vi "Process.vi"(8 "error in":errorcluster, 11 "Inst UI.TSL210":refnum<class "Inst UI.TSL210.lvclass">) -> (0 "error out":errorcluster, 3 "Inst UI.TSL210 out":refnum<class "Inst UI.TSL210.lvclass">)   [LabVIEW 2019, in "Inst UI.TSL210.lvclass"]
doc: "---------------------------------------------------------------\nJKI State Machine Objects™\nhttp://jki.net/state-machine-objects/\nCopyright (C) 2005-2015, JKI <info@jki.net>\nALL RIGHTS RESERVEDJKI State Machine Objects (SMO) 1.0.0.5\nJKI - JKI\nCopyright (c) 2016, JKI"
uses:
  Inst UI.TSL210.lvclass
  C:/Program Files (x86)/National Instruments/LabVIEW 2019/vi.lib/JKI/JKI SMO/SMO/SMO.lvclass
  C:/Program Files (x86)/National Instruments/LabVIEW 2019/user.lib/LevyLab/Instrument Framework/SMOs/Instrument UI/Instrument UI.lvclass
  C:/Program Files (x86)/National Instruments/LabVIEW 2019/vi.lib/JKI/JKI SMO/SMO.UI/SMO.UI.lvclass
  Inst.TSL210/Typedefs/Inst.TSL210.getAll--Cluster.ctl
  Inst.TSL210/Inst.TSL210.lvclass
  C:/Program Files (x86)/National Instruments/LabVIEW 2019/user.lib/LevyLab/Instrument Framework/SMOs/Instrument/Instrument.lvclass
  Inst UI.TSL210.UI--Cluster.ctl
  Inst.TSL210/Typedefs/Inst.TSL210.Configuration--Cluster.ctl
  <userlib>/LevyLab/Instrument Framework/SMOs/Configuration/Configuration.lvclass
  <userlib>/LevyLab/Instrument Framework/SMOs/RemoteControl/Typedefs/Message--Cluster.ctl
  <userlib>/LevyLab/Instrument Framework/SMOs/Instrument UI/Instrument UI.lvclass/Instrument UI.ctl
  Inst.TSL210/Inst.TSL210.lvclass/Inst.TSL210.ctl
  <vilib>/JKI/JKI SMO/SMO/SMO.lvclass/SMO.ctl
  <userlib>/LevyLab/Instrument Framework/SMOs/Configuration/Configuration.lvclass/Configuration.ctl
  <userlib>/LevyLab/Instrument Framework/SMOs/Instrument/Instrument.lvclass/Instrument.ctl
  <userlib>/LevyLab/Instrument Framework/SMOs/Instrument/Typedefs/Client Type--Enum.ctl
  09e9697b-516c-49fb-b2dc-692589121b6f.vi
  <vilib>/JKI/JKI SMO/SMO/Private/ReftoDVR--SMO.vi
  09e9697b-516c-49fb-b2dc-692589121b6f.vi/379bd6ed-7175-4835-90d5-280f41800e0e.vi
  09e9697b-516c-49fb-b2dc-692589121b6f.vi/379bd6ed-7175-4835-90d5-280f41800e0e.vi/7bfb9d26-19d0-4cd4-b030-48c854af821e.vi
  <userlib>/LevyLab/Instrument Framework/SMOs/Instrument/API/Send and Receive.vi
  09e9697b-516c-49fb-b2dc-692589121b6f.vi/379bd6ed-7175-4835-90d5-280f41800e0e.vi/d46e0d54-596d-480e-9b39-258cc9e52f4c.vi
  <userlib>/LevyLab/Instrument Framework/SMOs/Instrument/Private/Get Client Type.vi
  09e9697b-516c-49fb-b2dc-692589121b6f.vi/379bd6ed-7175-4835-90d5-280f41800e0e.vi/7bfb9d26-19d0-4cd4-b030-48c854af821e.vi/413d7368-8c72-40f9-a9e1-c9350bcdc852.vi
  09e9697b-516c-49fb-b2dc-692589121b6f.vi/379bd6ed-7175-4835-90d5-280f41800e0e.vi/7bfb9d26-19d0-4cd4-b030-48c854af821e.vi/bc459748-91b0-49f1-8512-5e73c8ffb289.vi
  09e9697b-516c-49fb-b2dc-692589121b6f.vi/379bd6ed-7175-4835-90d5-280f41800e0e.vi/d46e0d54-596d-480e-9b39-258cc9e52f4c.vi/af8ed217-f9ef-471c-b3eb-caab39959489.vi
  09e9697b-516c-49fb-b2dc-692589121b6f.vi/379bd6ed-7175-4835-90d5-280f41800e0e.vi/d46e0d54-596d-480e-9b39-258cc9e52f4c.vi/8d1c0661-ba5e-4a3a-852d-68d407e70a08.vi
  09e9697b-516c-49fb-b2dc-692589121b6f.vi/379bd6ed-7175-4835-90d5-280f41800e0e.vi/d46e0d54-596d-480e-9b39-258cc9e52f4c.vi/af8ed217-f9ef-471c-b3eb-caab39959489.vi/d0ebee8b-1f12-49bb-8058-086192fc38ca.vi
  09e9697b-516c-49fb-b2dc-692589121b6f.vi/379bd6ed-7175-4835-90d5-280f41800e0e.vi/d46e0d54-596d-480e-9b39-258cc9e52f4c.vi/af8ed217-f9ef-471c-b3eb-caab39959489.vi/26840459-4f5a-4133-bf65-9e6873a2309e.vi
  <userlib>/LevyLab/Instrument Framework/SMOs/Instrument/Private/Get RC Connection Status.vi
  <userlib>/LevyLab/Instrument Framework/SMOs/Instrument/API/Enum to String.vi
  <userlib>/LevyLab/Instrument Framework/SMOs/RemoteControl/API/Send and Receive.vi
  <vilib>/Utility/Data Type/Get Type Information.vi
  <vilib>/JDP Science/JSONtext/JSON text to Variant.vi
  <vilib>/JDP Science/JSONtext/Variant to JSON Text.vi
  <vilib>/National Instruments/GUID Generator/Guid Generator.vi
  <userlib>/LevyLab/Instrument Framework/SMOs/Instrument/Private/Instrument.MessageFromProcess.EventStructure.vi
  <userlib>/LevyLab/Instrument Framework/SMOs/Instrument/Instrument.lvclass
  <vilib>/JDP Science/JSONtext/LVClass Serializer/JSONtext LVClass Serializer.lvclass
  <userlib>/LevyLab/Instrument Framework/SMOs/Instrument UI/Instrument UI.lvclass
  <vilib>/JKI/JKI SMO/SMO/SMO.lvclass
  <vilib>/JKI/JKI SMO/SMO.UI/SMO.UI.lvclass
  <userlib>/LevyLab/Instrument Framework/SMOs/RemoteControl/RemoteControl.lvclass
  C:/Program Files (x86)/National Instruments/LabVIEW 2019/user.lib/LevyLab/Instrument Framework/Instrument Types/VSource/Instrument.VSource.lvclass
panel:
  in  "ACC":bool
  in  "COH":bool
  in  "LD":bool
  in  "Power":dbl min=0.0 max=10.0 step=0.001
  in  "Wavelength":dbl=1260.0 min=1260.0 max=1340.0 step=0.01
  out "FT":bool
  out "ACC":bool
  out "ATT":bool
  out "SystemBusy":bool
  out "CurrLimit":bool
  out "TempError":bool
  out "COH":bool
  out "LD":bool
  out "Power (mW)":dbl
  out "Wavelength (nm)":dbl
  in  "Parameter 2":string
  out "Numeric":u32
  in  "Set Parameter":bool
  in  "Parameter":dbl
  in  "STOP":bool
  # "WAVELENGTH (nm)"
  # "POWER (mW)"
  # "SMO UI Template"
  # "For instructions on how to use the JKI State Machine Objects, examples and video tutorials, visit:\nhttp://jki.net/state-machine-objects/\n\nJKI State Machine Objects™\nhttp://jki.net/state-machine-objects/\nCopyright (C) 2005-2015, JKI <info@jki.net>\nALL RIGHTS RESERVED"
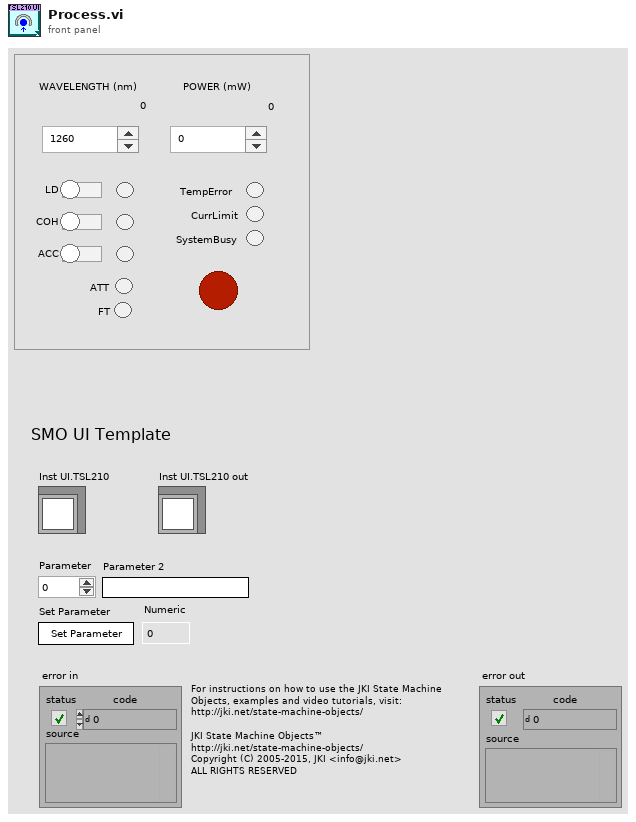
[diagram p1: front panel]
types:
  T1 = enum32{"invalid app kind", "Development System", "Run Time System", "Student Edition", "Embedded LabVIEW", "Evaluation", "Custom"}
  T2 = enum32{"Invalid", "Standard", "Closed", "Hidden", "Minimized", "Maximized"}
  T3 = typedef "Instrument.lvclass/Client Type--Enum.ctl" = enum16{"Remote", "Local"}
  T4 = typedef "Inst.TSL210.lvclass/Inst.TSL210.Configuration--Cluster.ctl" = cluster{"Example Setting":dbl}
  T5 = typedef "Inst.TSL210.lvclass/Inst.TSL210.getAll--Cluster.ctl" = cluster{"Wavelength (nm)":dbl, "Power (mW)":dbl, "Status: LD":bool, "Status: COH":bool, "Status: TempError":bool, "Status: CurrentLimit":bool, "Status: SystemBusy":bool, "Status: ATT":bool, "Status: ACC":bool, "Status: FT":bool}
  T6 = typedef "Inst UI.TSL210.lvclass/Inst UI.TSL210.UI--Cluster.ctl" = cluster{"Parameter":dbl, "Parameter 2":string}
  T7 = typedef "RemoteControl.lvclass/Message--Cluster.ctl" = cluster{"Command":string, "Data":variant, "ID":string}
  T8 = cluster{"Core":cluster{"Current VI Reference":refnum<vi>, "Close Panel on Exit?":bool, "Last Error":cluster{"error":errorcluster, "previous state":string, "remaining states":string}, "Shutdown?":bool}, "Instrument UI":refnum<class "Inst UI.TSL210.lvclass">, "Instrument":refnum<class "Inst.TSL210.lvclass">, "Configuration":refnum<class "Configuration.lvclass">, "Config Cluster":T4, "getAll":T5, "UI Cluster":T6, "Message":T7}
  T9 = cluster{"Current VI Reference":refnum<vi>, "Close Panel on Exit?":bool, "Last Error":cluster{"error":errorcluster, "previous state":string, "remaining states":string}, "Shutdown?":bool}
  T10 = typedef "SMO.lvclass/Protected Events.ctl" = cluster{"StopProcesses":refnum<user-event>, "AbortProcesses":refnum<user-event>, "Config Changed":refnum<user-event>, "Dependency":refnum<user-event>}
  T11 = typedef "Instrument.lvclass/PublicEvents--Cluster.ctl" = cluster{"MessageFromProcess":refnum<user-event>}
  T12 = typedef "Inst.TSL210.lvclass/PublicEvents--Cluster.ctl" = cluster{"MessageFromProcess":refnum<user-event>}
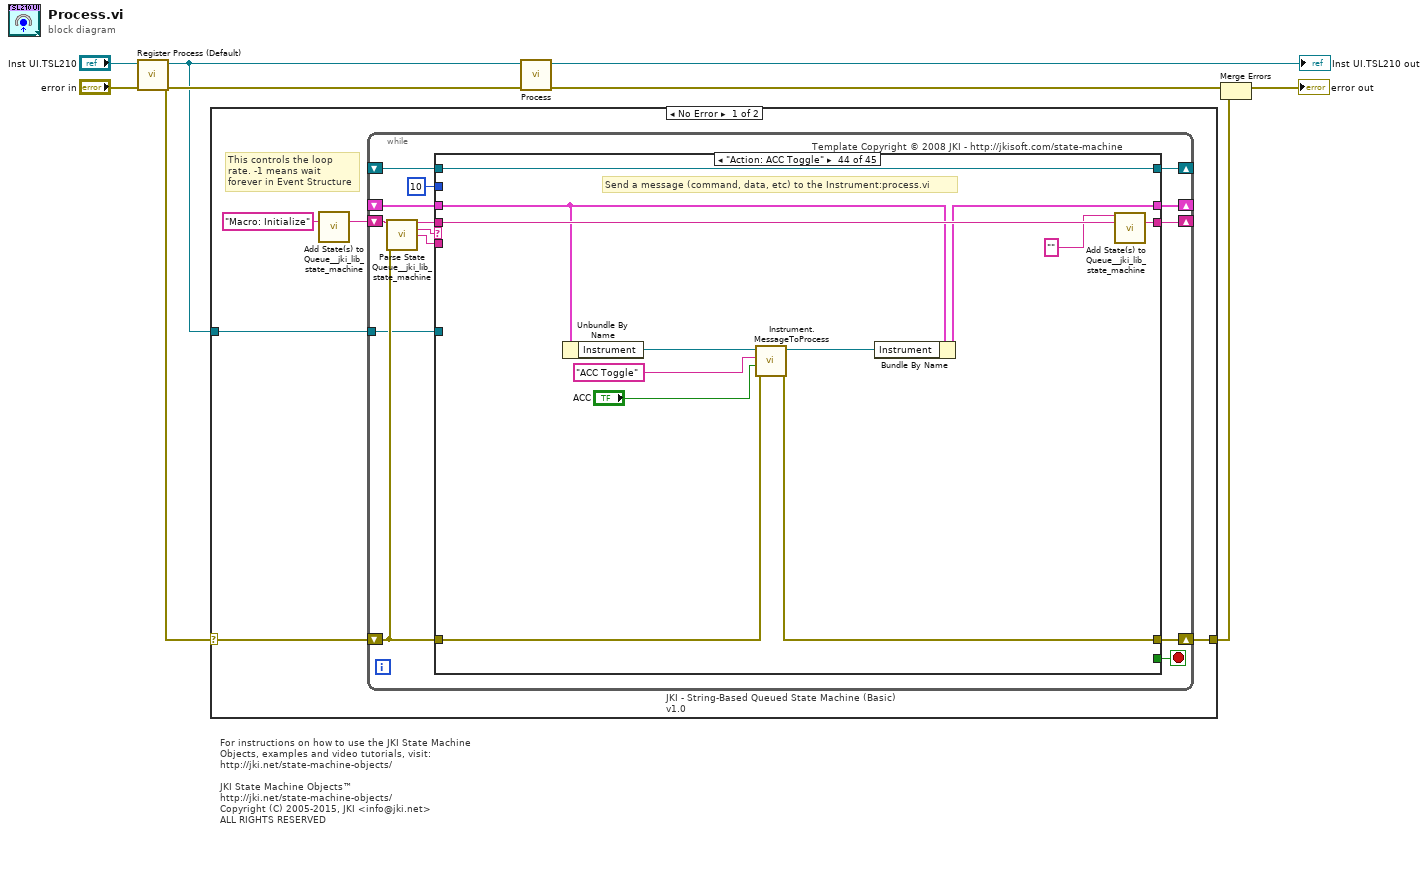
[diagram p0: block diagram]
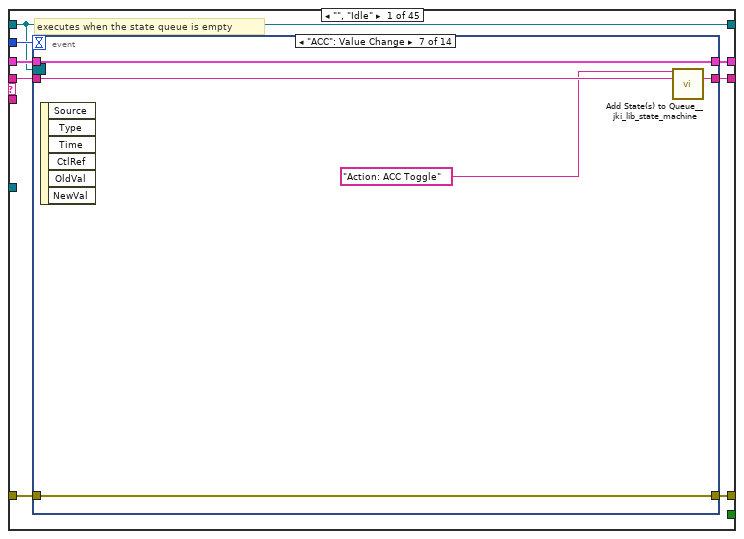
[diagram p2: hidden frame]
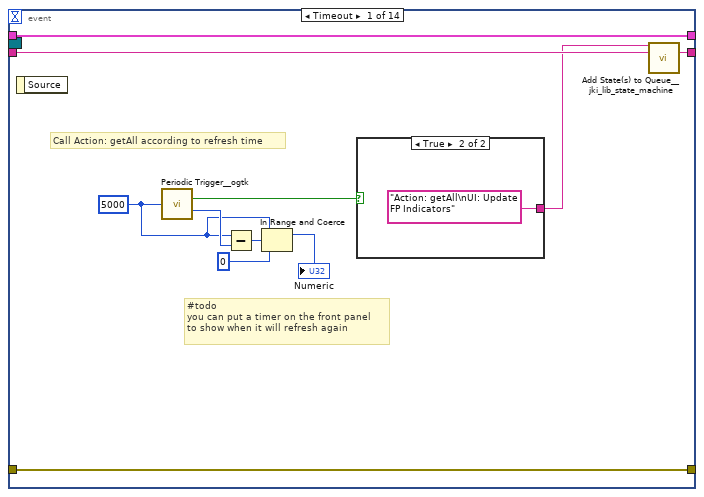
[diagram p3: hidden frame]
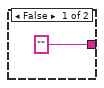
[diagram p4: hidden frame]
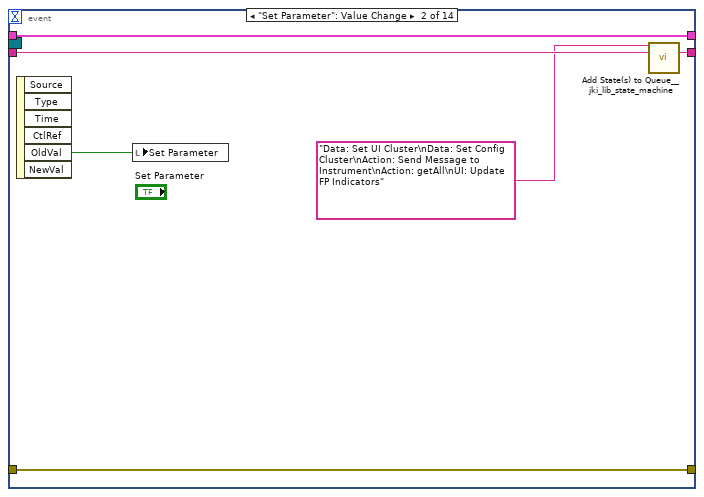
[diagram p5: hidden frame]
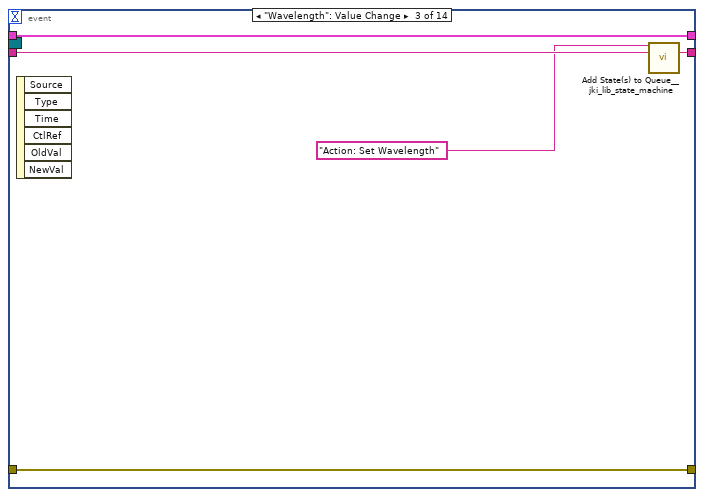
[diagram p6: hidden frame]
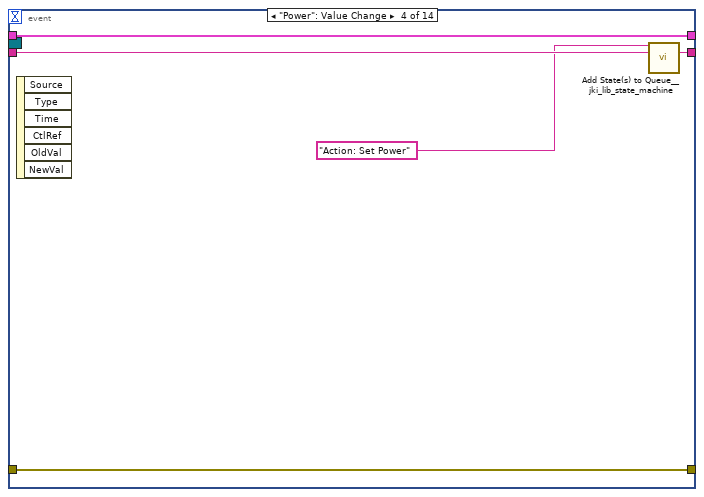
[diagram p7: hidden frame]
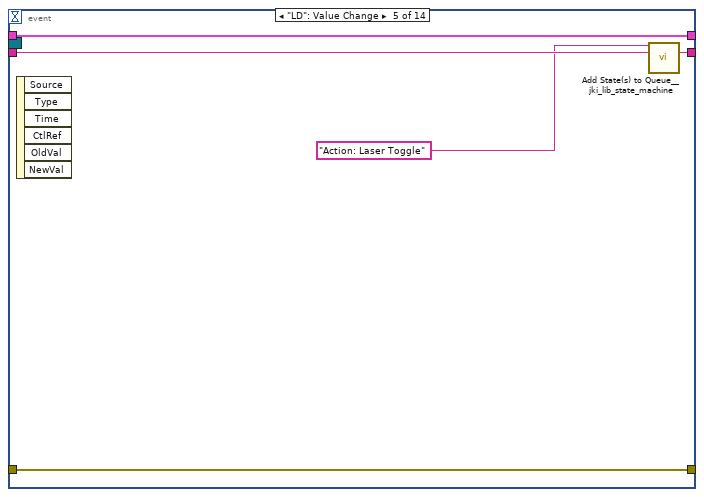
[diagram p8: hidden frame]
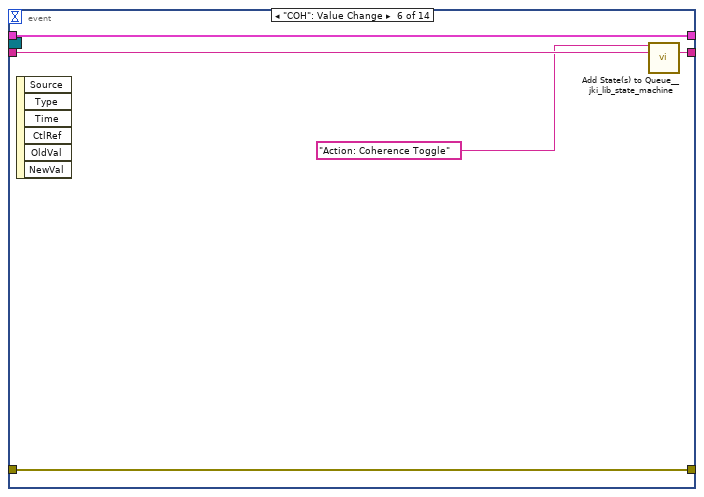
[diagram p9: hidden frame]
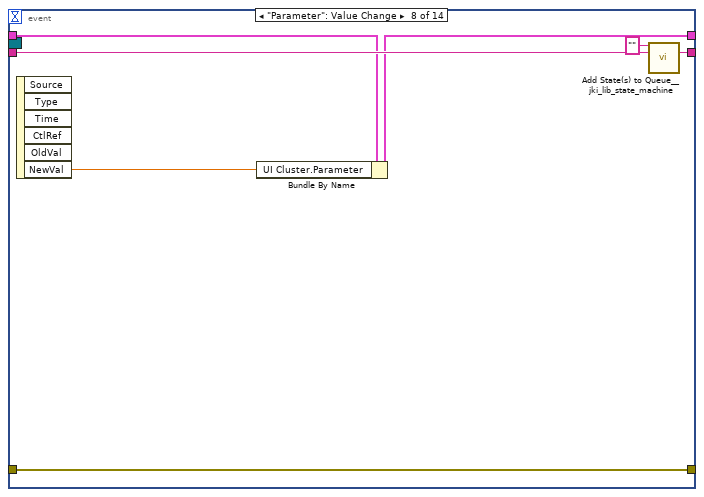
[diagram p10: hidden frame]
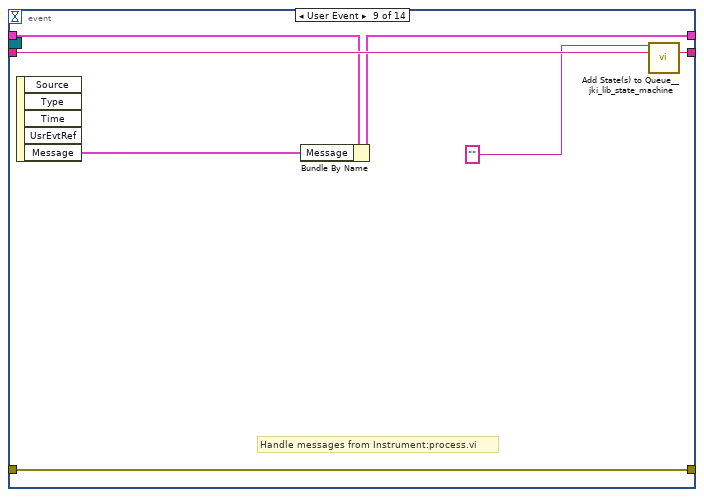
[diagram p11: hidden frame]
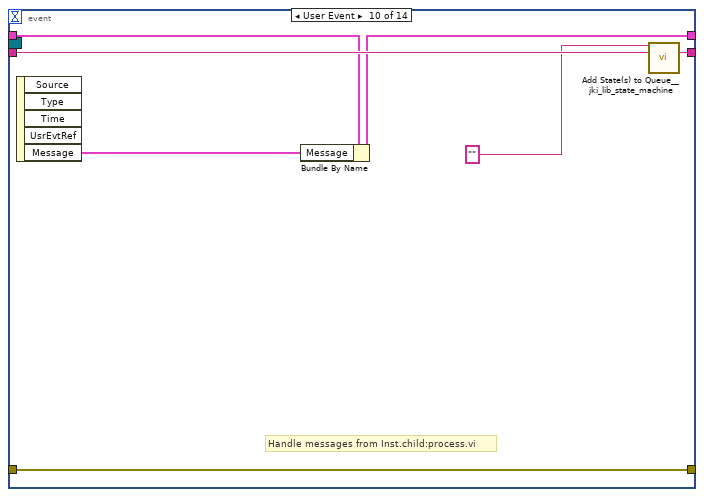
[diagram p12: hidden frame]
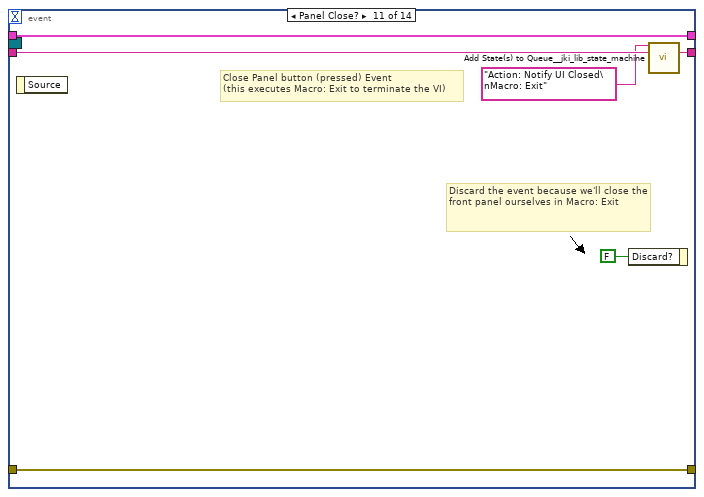
[diagram p13: hidden frame]
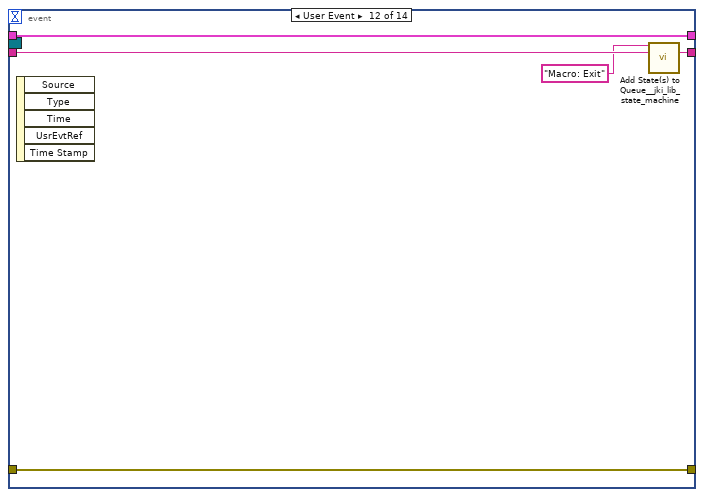
[diagram p14: hidden frame]
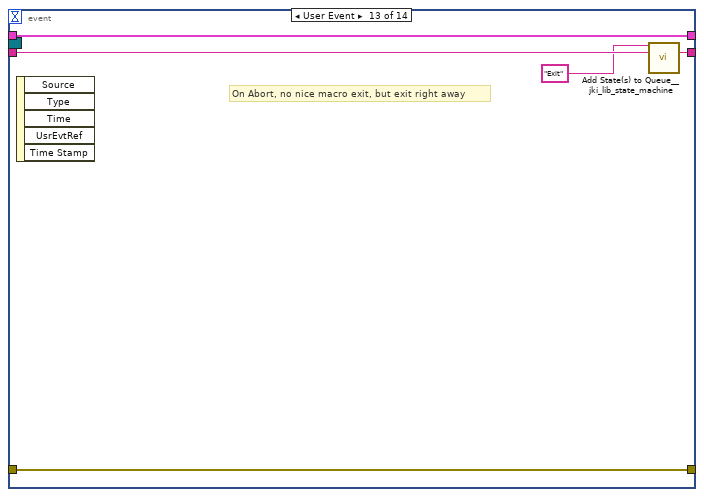
[diagram p15: hidden frame]
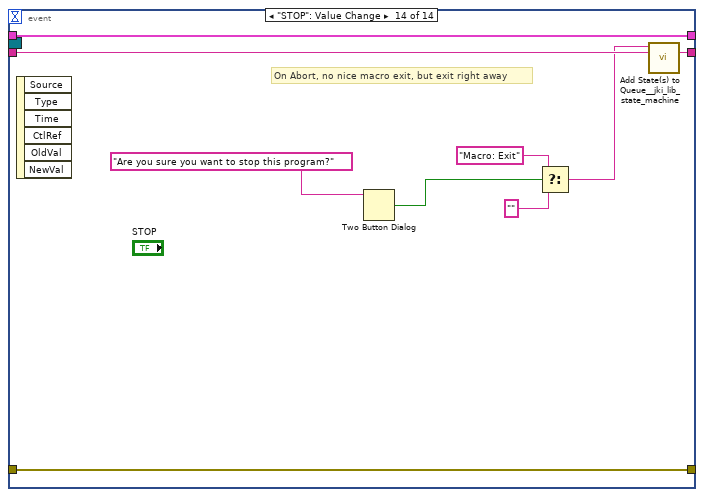
[diagram p16: hidden frame]
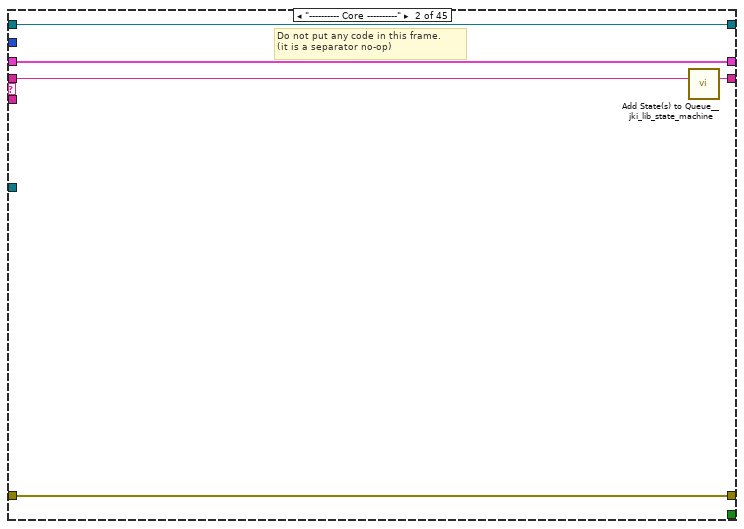
[diagram p17: hidden frame]
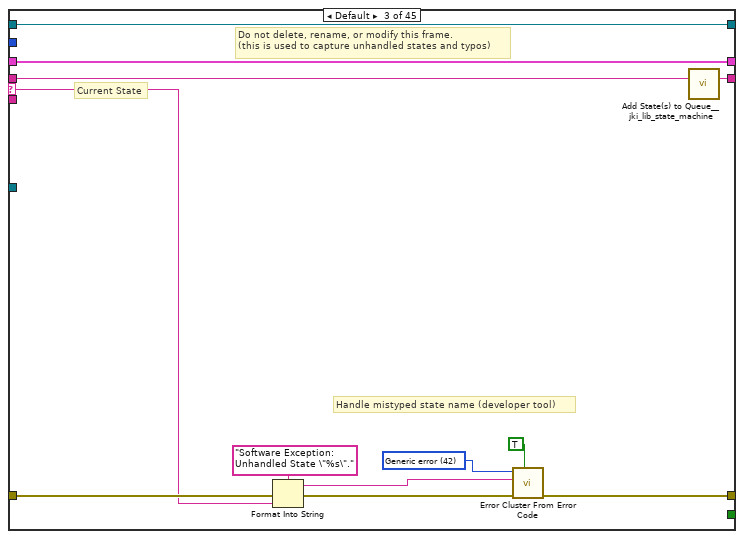
[diagram p18: hidden frame]
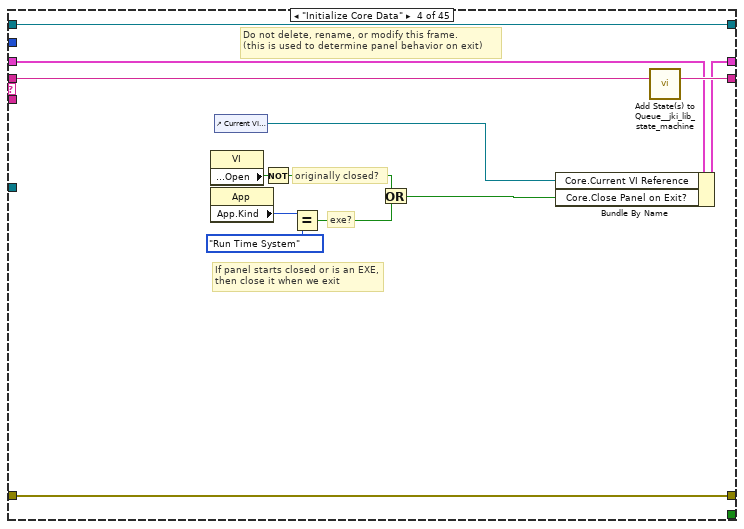
[diagram p19: hidden frame]
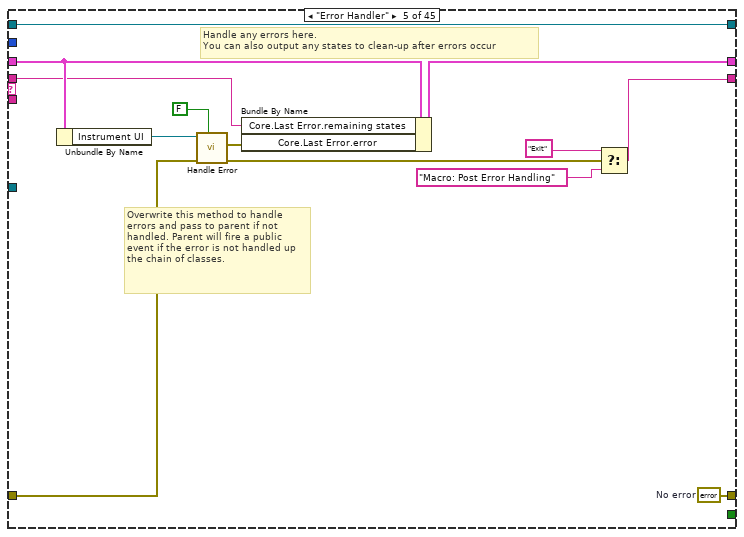
[diagram p20: hidden frame]
diagram:
  # "For instructions on how to use the JKI State Machine Objects, examples and video tutorials, visit:\nhttp://jki.net/state-machine-objects/\n\nJKI State Machine Objects™\nhttp://jki.net/state-machine-objects/\nCopyright (C) 2005-2015, JKI <info@jki.net>\nALL RIGHTS RESERVED"
  n1 = call <vilib>:"Register Process (Default).vi"("error in (no error)"="error in", "SMO"="Inst UI.TSL210") -> ("error out"=w5:errorcluster, "SelfRef"=w4:refnum<class "Inst UI.TSL210.lvclass">)  [unwired: 8 in]
  n2 = case shown="No Error" w5 {
    selector: w5 -> [w10 w579]
    tunnel: w4 -> [w11 _]
    tunnel: [w9 w579] -> w1
    frame No Error {
      # "This controls the loop rate. -1 means wait forever in Event Structure"
      n3 = call <vilib>:"Add State(s) to Queue__jki_lib_state_machine.vi"("State(s) in (\"\")"="Macro: Initialize") -> ("States Out"=w13:string)  [unwired: 14 in]
      n4 = while "JKI - String-Based Queued State Machine (Basic) v1.0" {
        shift-right: [w20] -> _
        shift-left: _ -> [w19]
        shift-right: [w23] -> w9
        shift-left: w10 -> [w17]
        shift-right: [w22] -> _
        shift-left: w13 -> [w24]
        tunnel: w11 -> [w16]
        shift-right: [w15] -> _
        shift-left: _ -> [w14]
        stop <- w21 stop-if-true
        # "Template Copyright © 2008 JKI - http://jkisoft.com/state-machine"
        n5 = call <vilib>:"Parse State Queue__jki_lib_state_machine.vi"("State Queue"=w24, "Error In (no error)"=w17) -> ("Remaining States"=w26:string, "Current State"=w27:string, "Arguments"=w25:string)  [unwired: 11 in]
        n6 = case shown="\"Action: ACC Toggle\"" w27 {
          selector: w27 -> [_ _ w132 _ _ _ _ _ _ _ _ _ _ _ _ _ _ _ _ _ _ _ _ _ _ _ _ _ _ _ _ _ _ _ _ _ _ _ _ _ _ _ _ _ _]
          tunnel: w26 -> [w35 w130 w136 w155 w159 w174 w179 w197 w205 w210 w217 w222 w229 w236 w252 w259 w275 w307 w316 w328 w338 w344 w359 w364 w375 w382 w387 w403 w409 w414 w429 w437 w449 w456 w463 w475 w488 w498 w508 w520 w532 w544 w556 w568 w578]
          tunnel: w25 -> [_ _ _ _ _ _ _ _ _ _ _ _ _ _ _ w253 w269 _ _ _ _ _ _ _ _ _ _ _ _ _ _ _ _ _ _ _ _ _ _ _ _ _ _ _ _]
          tunnel: w19 -> [w33 w127 w134 w146 w162 w170 w176 _ w201 w206 w211 w219 w227 w232 w247 w257 w271 w304 w312 w318 w335 w341 w346 w361 w372 w377 w384 w401 w407 w411 w422 w434 w440 w451 w457 w467 w482 w490 w503 w515 w527 w539 w551 w563 w573]
          tunnel: [w32 w128 w138 w152 w164 w169 w177 w184 w203 w208 w213 w220 w224 w234 w248 w254 w272 w305 w314 w326 w336 w342 w357 w362 w366 w378 w385 w398 w404 w412 w415 w432 w441 w453 w458 w472 w485 w495 w499 w511 w523 w535 w547 w559 w569] -> w23
          tunnel: w17 -> [w31 w128 w137 w152 w158 _ w177 w181 w203 w208 w214 w220 w225 w234 w248 w255 w273 w305 w314 w326 w336 w342 w357 w362 w367 w379 w385 w388 w405 w412 w424 w430 w442 w453 w459 w468 w477 w491 w500 w512 w524 w536 w548 w560 w570]
          tunnel: [w34 w129 w135 w154 w156 w173 w178 w196 w204 w209 w216 w221 w228 w235 w251 w258 w274 w306 w315 w327 w337 w343 w358 w363 w374 w381 w386 w402 w408 w413 w428 w436 w448 w455 w462 w474 w487 w497 w507 w519 w531 w543 w555 w567 w577] -> w22
          tunnel: [_ _ _ _ _ TRUE _ _ _ _ _ _ _ _ _ _ _ _ _ _ _ _ _ _ _ _ _ _ _ _ _ _ _ _ _ _ _ _ _ _ _ _ _ _ _] -> w21
          tunnel: [w30 w127 w134 w153 w161 w170 w176 w195 w200 w206 w211 w219 w227 w232 w247 w257 w271 w304 w312 w319 w335 w341 w346 w361 w372 w377 w384 w401 w407 w411 w426 w434 w438 w450 w457 w469 w483 w492 w504 w516 w528 w540 w552 w564 w574] -> w20
          tunnel: 10 ("Timeout") -> [w29 _ _ _ _ _ _ _ _ _ _ _ _ _ _ _ _ _ _ _ _ _ _ _ _ _ _ _ _ _ _ _ _ _ _ _ _ _ _ _ _ _ _ _ _]
          tunnel: w16 -> [_ _ _ _ _ _ _ w182 _ _ _ _ _ _ _ _ _ _ _ _ _ _ _ _ _ _ _ _ _ _ _ _ _ _ _ _ _ _ _ _ _ _ _ _ _]
          tunnel: [w28 w126 w131 w143 w168 w171 w175 w194 w202 w207 w212 w218 w226 w233 w250 w256 w268 w303 w313 w325 w334 w340 w351 w360 w373 w380 w383 w400 w406 w410 w427 w435 w447 w454 w461 w473 w486 w496 w506 w518 w530 w542 w554 w566 w576] -> w15
          tunnel: w14 -> [w28 w126 w131 w143 w168 w171 w175 w194 w202 w207 w212 w218 w226 w233 w250 w256 w268 w303 w313 w325 w334 w340 w351 w360 w373 w380 w383 _ w406 w410 w427 w435 w447 w454 w461 w473 w486 w496 w506 w518 w530 w542 w554 w566 w576]
          frame "", "Idle" {
            # "executes when the state queue is empty"
            n7 = event shown="[6] \"ACC\": Value Change" {
              selector: w28 -> [_ _ _ _ _ _ _ _ _ _ _ _ _ _]
              dyn-events: _ -> [_ _ _ _ _ _ _ _ _ _ _ _ _ _]
              timeout: w29 -> [_ _ _ _ _ _ _ _ _ _ _ _ _ _]
              tunnel: w35 -> [w46 w54 w59 w64 w69 w74 w79 w86 w93 w100 w106 w111 w116 w125]
              tunnel: [w45 w53 w58 w63 w68 w73 w78 w85 w92 w99 w105 w110 w115 w124] -> w34
              tunnel: w33 -> [w43 w51 w56 w61 w66 w71 w76 w82 w90 w97 w102 w108 w113 w122]
              tunnel: [w44 w52 w57 w62 w67 w72 w77 w84 w91 w98 w101 w109 w114 w123] -> w32
              tunnel: w31 -> [w44 w52 w57 w62 w67 w72 w77 w84 w91 w98 w101 w109 w114 w123]
              tunnel: [w43 w51 w56 w61 w66 w71 w76 w81 w89 w96 w102 w108 w113 w122] -> w30
              event Timeout {
                w37 = u32 5000 ("time (ms)")
                # "#todo\nyou can put a timer on the front panel\nto show when it will refresh again"
                # "Call Action: getAll according to refresh time"
                n8 = event-data() -> ()  [unwired: 1 in, 1 out]
                n9 = call <userlib>:"Periodic Trigger__ogtk.vi"("time (ms)"=w37) -> ("Triggered"=w41:bool, "timer value"=w40:u32)  [unwired: 12 in, 1 out]
                n10 = Subtract(x=w37, y=w40) -> (x-y=w39:u32)
                n11 = In Range and Coerce(upper limit=w37, x=w39, lower limit=u32 0) -> (coerced(x)=→"Numeric":u32)  [unwired: 1 out]
                n12 = case shown="True" w41 {
                  tunnel: ["" ("State(s) in Front (\"\")") "Action: getAll\nUI: Update FP Indicators" ("State(s) in Front (\"\")")] -> w42
                  frame False {
                  }
                  frame True {
                  }
                }
                n13 = call <vilib>:"Add State(s) to Queue__jki_lib_state_machine.vi"("State(s) in Front (\"\")"=w42, "State(s) in (\"\")"=w46) -> ("States Out"=w45:string)  [unwired: 13 in]
              }
              event "Set Parameter": Value Change {
                n14 = event-data() -> ("OldVal"=w50:bool)  [unwired: 1 in, 5 out]
                n15 = local write "Set Parameter"(w50) -> ()
                n16 = call <vilib>:"Add State(s) to Queue__jki_lib_state_machine.vi"("State(s) in Front (\"\")"="Data: Set UI Cluster\nData: Set Config Cluster\nAction: Send Message to Instrument\nAction: getAll\nUI: Update FP Indicators" ("State(s) in Front (\"\")"), "State(s) in (\"\")"=w54) -> ("States Out"=w53:string)  [unwired: 13 in]
              }
              event "Wavelength": Value Change {
                n17 = event-data() -> ()  [unwired: 1 in, 6 out]
                n18 = call <vilib>:"Add State(s) to Queue__jki_lib_state_machine.vi"("State(s) in Front (\"\")"="Action: Set Wavelength" ("State(s) in Front (\"\")"), "State(s) in (\"\")"=w59) -> ("States Out"=w58:string)  [unwired: 13 in]
              }
              event "Power": Value Change {
                n19 = event-data() -> ()  [unwired: 1 in, 6 out]
                n20 = call <vilib>:"Add State(s) to Queue__jki_lib_state_machine.vi"("State(s) in Front (\"\")"="Action: Set Power" ("State(s) in Front (\"\")"), "State(s) in (\"\")"=w64) -> ("States Out"=w63:string)  [unwired: 13 in]
              }
              event "LD": Value Change {
                n21 = event-data() -> ()  [unwired: 1 in, 6 out]
                n22 = call <vilib>:"Add State(s) to Queue__jki_lib_state_machine.vi"("State(s) in Front (\"\")"="Action: Laser Toggle" ("State(s) in Front (\"\")"), "State(s) in (\"\")"=w69) -> ("States Out"=w68:string)  [unwired: 13 in]
              }
              event "COH": Value Change {
                n23 = event-data() -> ()  [unwired: 1 in, 6 out]
                n24 = call <vilib>:"Add State(s) to Queue__jki_lib_state_machine.vi"("State(s) in Front (\"\")"="Action: Coherence Toggle" ("State(s) in Front (\"\")"), "State(s) in (\"\")"=w74) -> ("States Out"=w73:string)  [unwired: 13 in]
              }
              event "ACC": Value Change {
                n25 = event-data() -> ()  [unwired: 1 in, 6 out]
                n26 = call <vilib>:"Add State(s) to Queue__jki_lib_state_machine.vi"("State(s) in Front (\"\")"="Action: ACC Toggle" ("State(s) in Front (\"\")"), "State(s) in (\"\")"=w79) -> ("States Out"=w78:string)  [unwired: 13 in]
              }
              event "Parameter": Value Change {
                n27 = event-data() -> ("NewVal"=w83:dbl)  [unwired: 1 in, 5 out]
                n28 = Bundle By Name(cluster=w82, "UI Cluster.Parameter"=w83) -> (w81:T8)
                n29 = call <vilib>:"Add State(s) to Queue__jki_lib_state_machine.vi"("State(s) in Front (\"\")"="" ("State(s) in Front (\"\")"), "State(s) in (\"\")"=w86) -> ("States Out"=w85:string)  [unwired: 13 in]
              }
              event User Event {
                # "Handle messages from Instrument:process.vi"
                n30 = event-data() -> ("Message"=w87:T7)  [unwired: 1 in, 4 out]
                n31 = Bundle By Name(cluster=w90, "Message"=w87) -> (w89:T8)
                n32 = call <vilib>:"Add State(s) to Queue__jki_lib_state_machine.vi"("State(s) in Front (\"\")"="" ("State(s) in Front (\"\")"), "State(s) in (\"\")"=w93) -> ("States Out"=w92:string)  [unwired: 13 in]
              }
              event User Event {
                # "Handle messages from Inst.child:process.vi"
                n33 = event-data() -> ("Message"=w94:T7)  [unwired: 1 in, 4 out]
                n34 = Bundle By Name(cluster=w97, "Message"=w94) -> (w96:T8)
                n35 = call <vilib>:"Add State(s) to Queue__jki_lib_state_machine.vi"("State(s) in Front (\"\")"="" ("State(s) in Front (\"\")"), "State(s) in (\"\")"=w100) -> ("States Out"=w99:string)  [unwired: 13 in]
              }
              event Panel Close? {
                # "Discard the event because we'll close the front panel ourselves in Macro: Exit"
                # "Close Panel button (pressed) Event\n(this executes Macro: Exit to terminate the VI)"
                n36 = event-data() -> ()  [unwired: 1 in, 1 out]
                n37 = event-data("Discard?"=FALSE) -> ()  [unwired: 1 in, 1 out]
                n38 = call <vilib>:"Add State(s) to Queue__jki_lib_state_machine.vi"("State(s) in Front (\"\")"="Action: Notify UI Closed\nMacro: Exit", "State(s) in (\"\")"=w106) -> ("States Out"=w105:string)  [unwired: 13 in]
              }
              event User Event {
                n39 = event-data() -> ()  [unwired: 1 in, 5 out]
                n40 = call <vilib>:"Add State(s) to Queue__jki_lib_state_machine.vi"("State(s) in Front (\"\")"="Macro: Exit", "State(s) in (\"\")"=w111) -> ("States Out"=w110:string)  [unwired: 13 in]
              }
              event User Event {
                # "On Abort, no nice macro exit, but exit right away"
                n41 = event-data() -> ()  [unwired: 1 in, 5 out]
                n42 = call <vilib>:"Add State(s) to Queue__jki_lib_state_machine.vi"("State(s) in Front (\"\")"="Exit", "State(s) in (\"\")"=w116) -> ("States Out"=w115:string)  [unwired: 13 in]
              }
              event "STOP": Value Change {
                # "On Abort, no nice macro exit, but exit right away"
                n43 = event-data() -> ()  [unwired: 1 in, 6 out]
                n44 = Two Button Dialog(message="Are you sure you want to stop this program?") -> (T button?=w121:bool)  [unwired: 2 in]
                n45 = Select(t="Macro: Exit", s=w121, f="") -> (s? t:f=w117:string)
                n46 = call <vilib>:"Add State(s) to Queue__jki_lib_state_machine.vi"("State(s) in Front (\"\")"=w117, "State(s) in (\"\")"=w125) -> ("States Out"=w124:string)  [unwired: 13 in]
              }
            }
          }
          frame "---------- Core ----------" {
            # "Do not put any code in this frame.\n(it is a separator no-op)"
            n47 = call <vilib>:"Add State(s) to Queue__jki_lib_state_machine.vi"("State(s) in (\"\")"=w130) -> ("States Out"=w129:string)  [unwired: 14 in]
          }
          frame Default {
            w141 = 42 items=["No error", "Argument error", "Memory is full", "Out of zone", "End of file", "File already open", "Generic file I/O error", "File not found", "File permission error", "Disk is full", "Duplicate path", "Too many files open", "System feature not enabled", "Resource file not found", "Cannot add resource", "Resource not found", "Image not found", "Image memory error", "Pen does not exist", "Config type invalid", "Config token not found", "Config parse error", "Config memory error", "Bad external code format", "Bad external code offset", "External code not present", "Null window", "Destroy window error", "Null menu", "Print aborted", "Bad print record", "Print driver error", "Windows error during printing", "Memory error during printing", "Print dialog error", "Generic print error", "Invalid device refnum", "Device not found", "Device parameter error", "Device unit error", "Cannot open device", "Device call aborted", "Generic error", "Cancelled by user", "Object ID too low", "Object ID too high", "Object not in heap", "Unknown heap", "Unknown object (invalid DefProc)", "Unknown object (DefProc not in table)", "Message out of range", "Invalid (null) method", "Unknown message", "Manager call not supported", "Bad address", "Network operation in progress", "Network operation timed out", "Connection is busy", "Network attribute not supported", "Network error", "Address in use", "System out of memory", "Connection aborted", "Connection refused", "Not connected", "Already connected", "Connection closed", "Initialization error (interapplication manager)", "Bad occurrence", "Wait on unbound occurrence handler", "Occurrence queue overflow", "Datalog type conflict", "Unused", "Unrecognized type (interapplication manager)", "Memory corrupt", "Failed to make temporary DLL", "Old CIN version", "Drag socket not found", "Failed to load drop-object", "Failed to register OLE object", "Failed to release OLE object", "Format specifier type mismatch", "Unknown format specifier", "Too few format specifiers", "Too many format specifiers", "Scan failed", "Newer CIN version", "Error converting to variant", "Runtime menu error", "Password tampered", "Variant attribute not found", "Incompatible variant data type", "Event data is not available", "Event Store is not present", "Occurrence is not found", "Event Queue is not created", "Event info is not available", "Refnum passed is NULL", "Error retrieving Class GUID", "Error retrieving CoClass GUID", "Error retrieving TypeLib GUID.", "Bad built application magic bytes.", "Specific driver is different from the specific driver associated with the Logical Name.", "There is no session opened to the class driver.", "Max Error", "MAX - Error with config objects", "MAX - Error loading configuration", "MAX - Group not supported"]
            # "Current State"
            # "Do not delete, rename, or modify this frame.\n(this is used to capture unhandled states and typos)"
            # "Handle mistyped state name (developer tool)"
            n48 = Format Into String(format string="Software Exception: Unhandled State \"%s\"." ("message"), error in=w137, w132) -> (resulting string=w140:string, error out=w139:errorcluster)  [unwired: 1 in]
            n49 = call <vilib>:"Error Cluster From Error Code.vi"("show call chain? (False)"=TRUE, "error in (no error)"=w139, "error message (\"\")"=w140, "error code (0)"=w141) -> ("error out"=w138:errorcluster)  [unwired: 5 in]
            n50 = call <vilib>:"Add State(s) to Queue__jki_lib_state_machine.vi"("State(s) in (\"\")"=w136) -> ("States Out"=w135:string)  [unwired: 14 in]
          }
          frame "Initialize Core Data" {
            # "Do not delete, rename, or modify this frame.\n(this is used to determine panel behavior on exit)"
            # "originally closed?"
            # "exe?"
            # "If panel starts closed or is an EXE, then close it when we exit"
            n51 = property class="VI"() -> ("Front Panel.Open"=w151:bool)  [unwired: 2 in, 2 out]
            n52 = property class="App"() -> ("App.Kind"=w150:T1)  [unwired: 2 in, 2 out]
            n53 = control-ref of="Current VI Reference"() -> (w144:refnum<vi>)
            n54 = Not(x=w151) -> (.not. x?=w148:bool)
            n55 = Equal?(x=w150, y=T1."Run Time System" ("Application:Kind")) -> (x = y?=w147:bool)
            n56 = Or(x=w148, y=w147) -> (x .or. y?=w145:bool)
            n57 = Bundle By Name(cluster=w146, "Core.Current VI Reference"=w144, "Core.Close Panel on Exit?"=w145) -> (w153:T8)
            n58 = call <vilib>:"Add State(s) to Queue__jki_lib_state_machine.vi"("State(s) in (\"\")"=w155) -> ("States Out"=w154:string)  [unwired: 14 in]
          }
          frame "Error Handler" {
            w164 = errorcluster {"status"=FALSE, "code"=0, "source"=""}  # No error
            # "Overwrite this method to handle errors and pass to parent if not handled. Parent will fire a public event if the error is not handled up the chain of classes."
            # "Handle any errors here.\nYou can also output any states to clean-up after errors occur"
            n59 = Unbundle By Name(w162) -> ("Instrument UI"=w167:refnum<class "Inst UI.TSL210.lvclass">)
            n60 = call-dynamic "Handle Error.vi"("Stop on Unhandled Error (T)"=FALSE, "error in"=w158, "SMO"=w167) -> ("handling error"=w165:errorcluster, "Unhandled error"=w163:errorcluster)  [unwired: 6 in, 1 out]
            n61 = Bundle By Name(cluster=w162, "Core.Last Error.remaining states"=w159, "Core.Last Error.error"=w163) -> (w161:T8)
            n62 = Select(t="Exit", s=w165, f="Macro: Post Error Handling") -> (s? t:f=w156:string)
          }
          frame "Exit" {
            # "Do not put any code in this frame.\n(No errors that occur here will be handled.)"
            n63 = Unbundle By Name(w170) -> ("Core.Last Error.error"=w169:errorcluster)
            n64 = call <vilib>:"Add State(s) to Queue__jki_lib_state_machine.vi"("State(s) in (\"\")"=w174) -> ("States Out"=w173:string)  [unwired: 14 in]
          }
          frame "---------- Data ----------" {
            # "Do not put any code in this frame.\n(It is a separator no-op. You can make a copy of this frame to create a new Data frame)"
            n65 = call <vilib>:"Add State(s) to Queue__jki_lib_state_machine.vi"("State(s) in (\"\")"=w179) -> ("States Out"=w178:string)  [unwired: 14 in]
          }
          frame "Data: Initialize" {
            w180 = T7 {"Command"="", "Data"=variant, "ID"=""}  # Message
            w183 = refnum<class "Configuration.lvclass"> refnum  # Configuration
            w186 = T4 {"Example Setting"=0.0}  # Config Cluster
            w188 = T6 {"Parameter"=0.0, "Parameter 2"=""}  # UI Cluster
            w190 = refnum<class "Inst.TSL210.lvclass"> refnum  # Instrument
            w192 = T5 {"Wavelength (nm)"=0.0, "Power (mW)"=0.0, "Status: LD"=FALSE, "Status: COH"=FALSE, "Status: TempError"=FALSE, "Status: CurrentLimit"=FALSE, "Status: SystemBusy"=FALSE, "Status: ATT"=FALSE, "Status: ACC"=FALSE, "Status: FT"=FALSE}  # getAll
            w193 = T9 {"Current VI Reference"=refnum, "Close Panel on Exit?"=FALSE, "Last Error"={"error"={"status"=FALSE, "code"=0, "source"=""}, "previous state"="", "remaining states"=""}, "Shutdown?"=FALSE}  # Core
            # "typedef from Child Instrument"
            # "Cluster of UI\ninformation you\nwant to save/load"
            # "Child Instrument"
            # "typedef from Child Instrument"
            # "do not delete - used by framework"
            # "Data names and types of shift register data are defined by this bundle."
            # "Initialize the shift-register data, here.\n(data names are defined by what you wire into the bundle function)"
            n66 = call <userlib>:"Read Instrument.vi"("error in (no error)"=w181, "Instrument UI in"=w182) -> ("error out"=w187:errorcluster, "Instrument"=w189:refnum<class "Instrument.lvclass">, "Instrument UI"=w191:refnum<class "Inst UI.TSL210.lvclass">)  [unwired: 7 in]
            n67 = To More Specific Class(target class=w190, reference=w189, error in=w187) -> (specific class reference=w185:refnum<class "Inst.TSL210.lvclass">, error out=w184:errorcluster)
            n68 = Bundle("Core"=w193, "Instrument UI"=w191, "Instrument"=w185, "Configuration"=w183, "Config Cluster"=w186, "getAll"=w192, "UI Cluster"=w188, "Message"=w180) -> (w195:T8)  [unwired: 1 in]
            n69 = call <vilib>:"Add State(s) to Queue__jki_lib_state_machine.vi"("State(s) in (\"\")"=w197) -> ("States Out"=w196:string)  [unwired: 14 in]
          }
          frame "Data: Set UI Cluster" {
            # "Do not put any code in this frame.\n(It is a separator no-op. You can make a copy of this frame to create a new Data frame)"
            n70 = Bundle By Name(cluster=w201, "UI Cluster.Parameter"="Parameter", "UI Cluster.Parameter 2"="Parameter 2") -> (w200:T8)
            n71 = call <vilib>:"Add State(s) to Queue__jki_lib_state_machine.vi"("State(s) in (\"\")"=w205) -> ("States Out"=w204:string)  [unwired: 14 in]
          }
          frame "Data: Set Config Cluster" {
            # "Do not put any code in this frame.\n(It is a separator no-op. You can make a copy of this frame to create a new Data frame)"
            n72 = Unbundle By Name(w206) -> ()  [unwired: 2 out]
            n73 = call <vilib>:"Add State(s) to Queue__jki_lib_state_machine.vi"("State(s) in (\"\")"=w210) -> ("States Out"=w209:string)  [unwired: 14 in]
          }
          frame "Data: Cleanup" {
            # "Cleanup any data and references, here.\n(this is called automatically, by the Macro: Exit)"
            n74 = Unbundle By Name(w211) -> ("Core.Current VI Reference"=w215:refnum<vi>)
            n75 = Close Reference(reference=w215, error in (no error)=w214) -> (error out=w213:errorcluster)
            n76 = call <vilib>:"Add State(s) to Queue__jki_lib_state_machine.vi"("State(s) in (\"\")"=w217) -> ("States Out"=w216:string)  [unwired: 14 in]
          }
          frame "---------- UI ----------" {
            # "Do not put any code in this frame.\n(It is a separator no-op. You can make a copy of this frame to create a new UI frame)"
            n77 = call <vilib>:"Add State(s) to Queue__jki_lib_state_machine.vi"("State(s) in (\"\")"=w222) -> ("States Out"=w221:string)  [unwired: 14 in]
          }
          frame "UI: Initialize" {
            # "size window to decoration box on front panel"
            # "Initialize the User Interface, here.\n(this is called automatically, by the Macro: Init)"
            n78 = invoke on="STOP" class="Bool (strict)" method="Reinit To Default"() -> ()  [unwired: 3 in, 3 out]
            n79 = call <userlib>:"Fit VI window to Largest Dec__ogtk.vi"("error in (no error)"=w225, "border spacing (2 px)"=0) -> ("error out"=w224:errorcluster)  [unwired: 4 in, 1 out]
            n80 = call <vilib>:"Add State(s) to Queue__jki_lib_state_machine.vi"("State(s) in (\"\")"=w229) -> ("States Out"=w228:string)  [unwired: 14 in]
          }
          frame "UI: Update FP Controls" {
            # "Do not put any code in this frame.\n(It is a separator no-op. You can make a copy of this frame to create a new UI frame)"
            n81 = Unbundle By Name(w232) -> ("UI Cluster.Parameter"=w230:dbl, "UI Cluster.Parameter 2"=w231:string)
            n82 = local write "Parameter 2"(w231) -> ()
            n83 = local write "Parameter"(w230) -> ()
            n84 = call <vilib>:"Add State(s) to Queue__jki_lib_state_machine.vi"("State(s) in (\"\")"=w236) -> ("States Out"=w235:string)  [unwired: 14 in]
          }
          frame "UI: Update FP Indicators" {
            n85 = Unbundle By Name(w247) -> ("getAll"=w249:T5)
            n86 = Unbundle By Name(w249) -> ("Wavelength (nm)"=→"Wavelength (nm)":dbl, "Power (mW)"=→"Power (mW)":dbl, "Status: LD"=→"LD":bool, "Status: COH"=→"COH":bool, "Status: TempError"=→"TempError":bool, "Status: CurrentLimit"=→"CurrLimit":bool, "Status: SystemBusy"=→"SystemBusy":bool, "Status: ATT"=→"ATT":bool, "Status: ACC"=→"ACC":bool, "Status: FT"=→"FT":bool)
            n87 = call <vilib>:"Add State(s) to Queue__jki_lib_state_machine.vi"("State(s) in (\"\")"=w252) -> ("States Out"=w251:string)  [unwired: 14 in]
          }
          frame "UI: Cursor Set" {
            # "Argument"
            # "Initialize the User Interface, here.\n(this is called automatically, by the Macro: Init)"
            n88 = disable-structure shown="Default" {
              disable-tunnel: w255 -> [w260 w263]
              disable-tunnel: [w260 w262] -> w254
              disable-tunnel: w253 -> [_ w261]
              frame condition #0 {
              }
              frame condition #1 (active) {
                n89 = case shown="\"Busy\"" w261 {
                  tunnel: w263 -> [w265 w267]
                  tunnel: [w264 w266] -> w262
                  frame "Idle", Default {
                    n90 = call <vilib>:"Unset Busy.vi"("error in (no error)"=w265) -> ("error out"=w264:errorcluster)  [unwired: 10 in]
                  }
                  frame "Busy" {
                    n91 = call <vilib>:"Set Busy.vi"("error in (no error)"=w267) -> ("error out"=w266:errorcluster)  [unwired: 9 in, 1 out]
                  }
                }
              }
            }
            n92 = call <vilib>:"Add State(s) to Queue__jki_lib_state_machine.vi"("State(s) in (\"\")"=w259) -> ("States Out"=w258:string)  [unwired: 14 in]
          }
          frame "UI: Front Panel State" {
            # "Argument"
            # "Set Front Panel Open or Closed\n(Usage: \"UI: Front Panel State >> Open|Close\")"
            n93 = Unbundle By Name(w271) -> ("Core.Current VI Reference"=w270:refnum<vi>)
            n94 = disable-structure shown="Default" {
              disable-tunnel: w273 -> [w279 w302]
              disable-tunnel: [w278 w302] -> w272
              disable-tunnel: w270 -> [w277 _]
              disable-tunnel: w269 -> [w276 _]
              frame condition #0 (active) {
                n95 = case shown="\"Close\"" w276 {
                  tunnel: w279 -> [w283 w296]
                  tunnel: [w285 w297] -> w278
                  tunnel: w277 -> [w284 w294]
                  frame "Open", Default {
                    n96 = property class="VI"(reference=w284, error in=w283) -> (reference out=w281:refnum<vi>, error out=w282:errorcluster, "FP.State"=w280:T2)
                    n97 = case shown="\"Closed\"" w280 {
                      tunnel: [w288 w291] -> w285
                      tunnel: w282 -> [w287 w291]
                      tunnel: w281 -> [w286 _]
                      frame "Closed" {
                        n98 = invoke class="VI" method="FP.Open"(reference=w286, error in=w287, "Activate"=TRUE, "State"=T2."Standard") -> (error out=w288:errorcluster)  [unwired: 1 in, 4 out]
                      }
                      frame Default {
                      }
                    }
                  }
                  frame "Close" {
                    n99 = property class="VI"(reference=w294, error in=w296) -> (reference out=w293:refnum<vi>, error out=w295:errorcluster, "FP.State"=w292:T2)
                    n100 = case shown="Default" w292 {
                      tunnel: [w298 w301] -> w297
                      tunnel: w295 -> [w298 w300]
                      tunnel: w293 -> [_ w299]
                      frame "Invalid", "Closed" {
                      }
                      frame Default {
                        n101 = invoke class="VI" method="FP.Close"(reference=w299, error in=w300) -> (error out=w301:errorcluster)  [unwired: 1 in, 2 out]
                      }
                    }
                  }
                }
              }
              frame condition #1 {
              }
            }
            n102 = call <vilib>:"Add State(s) to Queue__jki_lib_state_machine.vi"("State(s) in (\"\")"=w275) -> ("States Out"=w274:string)  [unwired: 14 in]
          }
          frame "---------- Macro ----------" {
            # "Do not put any code in this frame.\n(It is a separator no-op. You can make a copy of this frame to create a new Macro frame)"
            n103 = call <vilib>:"Add State(s) to Queue__jki_lib_state_machine.vi"("State(s) in (\"\")"=w307) -> ("States Out"=w306:string)  [unwired: 14 in]
          }
          frame "Macro: Initialize" {
            w310 = "UI: Initialize\nMacro: Read UI Config\nAction: Open\n//UI: Front Panel State >> Open"  # UI: Initialize Macro: Read UI Config Action: Open //UI: Front Panel State >> Open
            # "Initialization Macro\n(This is called once, when the VI starts)"
            n104 = call <vilib>:"Add State(s) to Queue__jki_lib_state_machine.vi"("State(s) in Front (\"\")"="Data: Initialize\nInitialize Core Data\nEvents: Register", "State(s) in (\"\")"="Process: Sync", "State(s) at Back (\"\")"=w310) -> ("States Out"=w309:string)  [unwired: 12 in]
            n105 = call <vilib>:"Add State(s) to Queue__jki_lib_state_machine.vi"("State(s) in Front (\"\")"=w309, "State(s) in (\"\")"=w316) -> ("States Out"=w315:string)  [unwired: 13 in]
          }
          frame "Macro: Post Error Handling" {
            # "Clear Last Error?"
            n106 = Unbundle By Name(w318) -> ("Core.Last Error.remaining states"=w320:string, "Core.Shutdown?"=w321:bool)
            n107 = Unbundle By Name(w318) -> ("Core.Last Error.error"=w324:errorcluster)
            n108 = case shown="False" FALSE {
              tunnel: w324 -> [w332 _]
              tunnel: [w332 _] -> w323
              frame False {
              }
              frame True {
              }
            }
            n109 = case shown="True" w321 {
              tunnel: w320 -> [w329 w331]
              tunnel: [w329 w330] -> w317
              frame False {
                # "These are the remaining states (at the moment the error occured). States can be altered according to business logic."
                # "NOT SHUTTING DOWN"
              }
              frame True {
                # "Developer can decide to alter the states but should be aware that during the shutdown process, there are certain states that must be run for the SMO to properly shut itself (and this process) down. As such, one can add states to perform additional clean-ups, but should append the remaining state to be executed."
                # "SHUTTING DOWN"
                n110 = call <vilib>:"Add State(s) to Queue__jki_lib_state_machine.vi"("State(s) in (\"\")"=w331) -> ("States Out"=w330:string)  [unwired: 14 in]
              }
            }
            n111 = Bundle By Name(cluster=w318, "Core.Last Error.error"=w323) -> (w319:T8)
            n112 = call <vilib>:"Add State(s) to Queue__jki_lib_state_machine.vi"("State(s) in Front (\"\")"=w317, "State(s) in (\"\")"=w328) -> ("States Out"=w327:string)  [unwired: 13 in]
          }
          frame "Macro: Read UI Config" {
            # "Do not put any code in this frame.\n(It is a separator no-op. You can make a copy of this frame to create a new Macro frame)"
            n113 = call <vilib>:"Add State(s) to Queue__jki_lib_state_machine.vi"("State(s) in Front (\"\")"="Configuration: Initialize\nConfiguration: Read UI Config File\nUI: Update FP Controls" ("State(s) in Front (\"\")"), "State(s) in (\"\")"=w338) -> ("States Out"=w337:string)  [unwired: 13 in]
          }
          frame "Macro: Write UI Config" {
            # "Do not put any code in this frame.\n(It is a separator no-op. You can make a copy of this frame to create a new Macro frame)"
            n114 = call <vilib>:"Add State(s) to Queue__jki_lib_state_machine.vi"("State(s) in Front (\"\")"="Data: Set UI Cluster\nConfiguration: Write UI Config File" ("State(s) in Front (\"\")"), "State(s) in (\"\")"=w344) -> ("States Out"=w343:string)  [unwired: 13 in]
          }
          frame "Macro: Exit" {
            # "Exit Macro\n(This is called once, when the VI exits)"
            n115 = Unbundle By Name(w346) -> ("Core.Close Panel on Exit?"=w356:bool)
            n116 = Select(t="UI: Front Panel State >> Close", s=w356, f="" ("Empty String Constant")) -> (s? t:f=w353:string)
            n117 = call <vilib>:"Add State(s) to Queue__jki_lib_state_machine.vi"("State(s) in Front (\"\")"="Data: Cleanup\nEvents: Unregister\nProcess: Self Terminate", "State(s) in (\"\")"="Process: Sync", "State(s) at Back (\"\")"="Exit") -> ("States Out"=w348:string)  [unwired: 12 in]
            n118 = call <vilib>:"Add State(s) to Queue__jki_lib_state_machine.vi"("State(s) in Front (\"\")"="Action: Close\nMacro: Write UI Config", "State(s) in (\"\")"=w353, "State(s) at Back (\"\")"=w348) -> ("States Out"=w352:string)  [unwired: 12 in]
            n119 = call <vilib>:"Add State(s) to Queue__jki_lib_state_machine.vi"("State(s) in Front (\"\")"=w352, "State(s) in (\"\")"=w359) -> ("States Out"=w358:string)  [unwired: 13 in]
          }
          frame "---------- Process ----------" {
            # "Template Separator\n(You can make a copy of, or modify, this frame)"
            n120 = call <vilib>:"Add State(s) to Queue__jki_lib_state_machine.vi"("State(s) in (\"\")"=w364) -> ("States Out"=w363:string)  [unwired: 14 in]
          }
          frame "Process: Sync" {
            n121 = Unbundle By Name(w372) -> ("Instrument UI"=w368:refnum<class "Inst UI.TSL210.lvclass">)
            n122 = call <vilib>:"WaitOnProcessSync.vi"("error in (no error)"=w367, "SMO"=w368) -> ("error out"=w366:errorcluster, "Don't run?"=w371:bool)  [unwired: 7 in, 1 out]
            n123 = Select(t="Data: Cleanup\nEvents: Unregister\nExit", s=w371, f="" ("Empty String Constant")) -> (s? t:f=w365:string)
            n124 = call <vilib>:"Add State(s) to Queue__jki_lib_state_machine.vi"("State(s) in Front (\"\")"=w365, "State(s) in (\"\")"=w375) -> ("States Out"=w374:string)  [unwired: 13 in]
          }
          frame "Process: Self Terminate" {
            n125 = Unbundle By Name(w377) -> ("Instrument UI"=w376:refnum<class "Inst UI.TSL210.lvclass">)
            n126 = call <vilib>:"SelfTerminate.vi"("error in (no error)"=w379, "SMO in"=w376) -> ("error out"=w378:errorcluster)  [unwired: 8 in, 1 out]
            n127 = call <vilib>:"Add State(s) to Queue__jki_lib_state_machine.vi"("State(s) in (\"\")"=w382) -> ("States Out"=w381:string)  [unwired: 14 in]
          }
          frame "---------- Events ----------" {
            # "Template Separator\n(You can make a copy of, or modify, this frame)"
            n128 = call <vilib>:"Add State(s) to Queue__jki_lib_state_machine.vi"("State(s) in (\"\")"=w387) -> ("States Out"=w386:string)  [unwired: 14 in]
          }
          frame "Events: Register" {
            # "Expand to add\nmore events"
            # "Base Class Protected Events"
            n129 = Unbundle By Name(w401) -> ("Instrument UI"=w394:refnum<class "Inst UI.TSL210.lvclass">, "Instrument"=w393:refnum<class "Inst.TSL210.lvclass">)
            n130 = call <vilib>:"GetProtectedEvents.vi"("SMO"=w394) -> ("error out"=w397:errorcluster, "SMO Protected Events"=w399:T10)  [unwired: 8 in, 1 out]
            n131 = call <userlib>:"Instrument.GetPublicEvents.vi"("Instrument"=w393) -> ("error out"=w395:errorcluster, "Instrument Public Events"=w396:T11, "Instrument out"=w391:refnum<class "Inst.TSL210.lvclass">)  [unwired: 8 in]
            n132 = call "Inst.TSL210.GetPublicEvents.vi"("Inst.TSL210 in"=w391) -> ("error out"=w390:errorcluster, "Inst.TSL210 Public Events"=w392:T12)  [unwired: 8 in, 1 out]
            n133 = register-events(w399, w396, w392) -> (reference out=w400:refnum<event-registration>, error out=w389:errorcluster)  [unwired: 2 in]
            n134 = Merge Errors(w389, w390, w395, w397, w388) -> (w398:errorcluster)
            n135 = call <vilib>:"Add State(s) to Queue__jki_lib_state_machine.vi"("State(s) in (\"\")"=w403) -> ("States Out"=w402:string)  [unwired: 14 in]
          }
          frame "Events: Unregister" {
            n136 = Unregister For Events(event registration refnum=w406, error in=w405) -> (error out=w404:errorcluster)
            n137 = call <vilib>:"Add State(s) to Queue__jki_lib_state_machine.vi"("State(s) in (\"\")"=w409) -> ("States Out"=w408:string)  [unwired: 14 in]
          }
          frame "---------- Configuration ----------" {
            # "Do not put any code in this frame.\n(It is a separator no-op. You can make a copy of this frame to create a new UI frame)"
            n138 = call <vilib>:"Add State(s) to Queue__jki_lib_state_machine.vi"("State(s) in (\"\")"=w414) -> ("States Out"=w413:string)  [unwired: 14 in]
          }
          frame "Configuration: Initialize" {
            # "Do not put any code in this frame.\n(It is a separator no-op. You can make a copy of this frame to create a new UI frame)"
            n139 = Unbundle By Name(w422) -> ("Configuration"=w420:refnum<class "Configuration.lvclass">, "Instrument"=w421:refnum<class "Inst.TSL210.lvclass">)
            n140 = call <vilib>:"GetName.vi"("error in (no error)"=w424, "SMO"=w421) -> ("error out"=w423:errorcluster, "Name"=w425:string)  [unwired: 6 in, 2 out]
            n141 = call <userlib>:"Default Path.vi"("error in (no error)"=w423, "Folder Name [Application Name]"=w425, "Configuration in"=w420) -> ("error out"=w416:errorcluster, "Configuration out"=w419:refnum<class "Configuration.lvclass">)  [unwired: 7 in]
            n142 = call <userlib>:"Write Section.vi"("error in (no error)"=w416, "Section"="UI", "Configuration in"=w419) -> ("error out"=w415:errorcluster, "Configuration out"=w418:refnum<class "Configuration.lvclass">)  [unwired: 7 in]
            n143 = Bundle By Name(cluster=w422, "Configuration"=w418) -> (w426:T8)
            n144 = call <vilib>:"Add State(s) to Queue__jki_lib_state_machine.vi"("State(s) in (\"\")"=w429) -> ("States Out"=w428:string)  [unwired: 14 in]
          }
          frame "Configuration: Write UI Config File" {
            # "Do not put any code in this frame.\n(It is a separator no-op. You can make a copy of this frame to create a new Data frame)"
            n145 = Unbundle By Name(w434) -> ("Configuration"=w431:refnum<class "Configuration.lvclass">, "UI Cluster"=w433:T6)
            n146 = call <userlib>:"Write Configuration.vi"("error in (no error)"=w430, "Variant"=w433, "Configuration in"=w431) -> ("error out"=w432:errorcluster)  [unwired: 7 in, 1 out]
            n147 = call <vilib>:"Add State(s) to Queue__jki_lib_state_machine.vi"("State(s) in (\"\")"=w437) -> ("States Out"=w436:string)  [unwired: 14 in]
          }
          frame "Configuration: Read UI Config File" {
            # "Do not put any code in this frame.\n(It is a separator no-op. You can make a copy of this frame to create a new UI frame)"
            n148 = Unbundle By Name(w440) -> ("UI Cluster"=w443:T6, "Configuration"=w446:refnum<class "Configuration.lvclass">)
            n149 = call <userlib>:"Read Configuration.vi"("INI Fomatted Cluster Type"=w443, "error in (no error)"=w442, "Configuration in"=w446) -> ("error out"=w445:errorcluster, "Configuration"=w444:variant)  [unwired: 6 in, 1 out]
            n150 = Variant To Data(error in=w445, type=w443, Variant=w444) -> (data=w439:T6, error out=w441:errorcluster)
            n151 = Bundle By Name(cluster=w440, "UI Cluster"=w439) -> (w438:T8)
            n152 = call <vilib>:"Add State(s) to Queue__jki_lib_state_machine.vi"("State(s) in (\"\")"=w449) -> ("States Out"=w448:string)  [unwired: 14 in]
          }
          frame "---------- Action ----------" {
            n153 = Unbundle By Name(w451) -> ("Instrument"=w452:refnum<class "Inst.TSL210.lvclass">)
            n154 = Bundle By Name(cluster=w451, "Instrument"=w452) -> (w450:T8)
            n155 = call <vilib>:"Add State(s) to Queue__jki_lib_state_machine.vi"("State(s) in (\"\")"=w456) -> ("States Out"=w455:string)  [unwired: 14 in]
          }
          frame "Action: Notify UI Closed" {
            # "Notify that the UI has been closed"
            n156 = Unbundle By Name(w457) -> ("Instrument UI"=w460:refnum<class "Inst UI.TSL210.lvclass">)
            n157 = call <vilib>:"Hide.vi"("error in (no error)"=w459, "SMO.UI"=w460) -> ("error out"=w458:errorcluster)  [unwired: 8 in, 1 out]
            n158 = call <vilib>:"Add State(s) to Queue__jki_lib_state_machine.vi"("State(s) in (\"\")"=w463) -> ("States Out"=w462:string)  [unwired: 14 in]
          }
          frame "Action: getAll" {
            n159 = Unbundle By Name(w467) -> ("getAll"=w465:T5, "Instrument"=w470:refnum<class "Inst.TSL210.lvclass">)
            n160 = call "GET ALL.vim"("type"=w465, "error in (no error)"=w468, "Instrument in"=w470) -> ("error out"=w472:errorcluster, "getAll"=w464:T5, "Instrument out"=w466:refnum<class "Inst.TSL210.lvclass">)  [unwired: 6 in]
            n161 = Bundle By Name(cluster=w467, "Instrument"=w466, "getAll"=w464) -> (w469:T8)
            n162 = call <vilib>:"Add State(s) to Queue__jki_lib_state_machine.vi"("State(s) in Front (\"\")"="" ("State(s) in Front (\"\")"), "State(s) in (\"\")"=w475) -> ("States Out"=w474:string)  [unwired: 13 in]
          }
          frame "Action: Open" {
            n163 = Unbundle By Name(w482) -> ("Instrument"=w480:refnum<class "Inst.TSL210.lvclass">)
            n164 = call <userlib>:"Write Client Type.vi"("error in (no error)"=w477, "Client Type"=Client_Type--Enum."Local", "Instrument in"=w480) -> ("error out"=w478:errorcluster, "Instrument out"=w479:refnum<class "Inst.TSL210.lvclass">)  [unwired: 7 in]
            n165 = call-dynamic "Open.vi"("error in (no error)"=w478, "Inst.TSL210 in"=w479) -> ("error out"=w485:errorcluster, "Inst.TSL210 out"=w481:refnum<class "Inst.TSL210.lvclass">)  [unwired: 8 in]
            n166 = Bundle By Name(cluster=w482, "Instrument"=w481) -> (w483:T8)
            n167 = call <vilib>:"Add State(s) to Queue__jki_lib_state_machine.vi"("State(s) in Front (\"\")"="" ("State(s) in Front (\"\")"), "State(s) in (\"\")"=w488) -> ("States Out"=w487:string)  [unwired: 13 in]
          }
          frame "Action: Close" {
            n168 = Unbundle By Name(w490) -> ("Instrument"=w493:refnum<class "Inst.TSL210.lvclass">)
            n169 = call-dynamic "Close.vi"("error in (no error)"=w491, "Inst.TSL210 in"=w493) -> ("error out"=w495:errorcluster, "Inst.TSL210 out"=w489:refnum<class "Inst.TSL210.lvclass">)  [unwired: 8 in]
            n170 = Bundle By Name(cluster=w490, "Instrument"=w489) -> (w492:T8)
            n171 = call <vilib>:"Add State(s) to Queue__jki_lib_state_machine.vi"("State(s) in Front (\"\")"="" ("State(s) in Front (\"\")"), "State(s) in (\"\")"=w498) -> ("States Out"=w497:string)  [unwired: 13 in]
          }
          frame "Action: Send Message to Instrument" {
            # "Send a message (command, data, etc) to the Instrument:process.vi"
            n172 = Unbundle By Name(w503) -> ("Instrument"=w502:refnum<class "Inst.TSL210.lvclass">)  [unwired: 1 out]
            n173 = call <userlib>:"Instrument.MessageToProcess.vi"("error in (no error)"=w500, "Instrument"=w502) -> ("error out"=w499:errorcluster, "Instrument out"=w501:refnum<class "Inst.TSL210.lvclass">)  [unwired: 8 in]
            n174 = Bundle By Name(cluster=w503, "Instrument"=w501) -> (w504:T8)
            n175 = call <vilib>:"Add State(s) to Queue__jki_lib_state_machine.vi"("State(s) in Front (\"\")"="" ("State(s) in Front (\"\")"), "State(s) in (\"\")"=w508) -> ("States Out"=w507:string)  [unwired: 13 in]
          }
          frame "Action: Set Wavelength" {
            # "Send a message (command, data, etc) to the Instrument:process.vi"
            n176 = Unbundle By Name(w515) -> ("Instrument"=w514:refnum<class "Inst.TSL210.lvclass">)
            n177 = call <userlib>:"Instrument.MessageToProcess.vi"("error in (no error)"=w512, "Data"="Wavelength", "Command"="Set Wavelength", "Instrument"=w514) -> ("error out"=w511:errorcluster, "Instrument out"=w513:refnum<class "Inst.TSL210.lvclass">)  [unwired: 6 in]
            n178 = Bundle By Name(cluster=w515, "Instrument"=w513) -> (w516:T8)
            n179 = call <vilib>:"Add State(s) to Queue__jki_lib_state_machine.vi"("State(s) in Front (\"\")"="" ("State(s) in Front (\"\")"), "State(s) in (\"\")"=w520) -> ("States Out"=w519:string)  [unwired: 13 in]
          }
          frame "Action: Set Power" {
            # "Send a message (command, data, etc) to the Instrument:process.vi"
            n180 = Unbundle By Name(w527) -> ("Instrument"=w526:refnum<class "Inst.TSL210.lvclass">)
            n181 = call <userlib>:"Instrument.MessageToProcess.vi"("error in (no error)"=w524, "Data"="Power", "Command"="Set Power", "Instrument"=w526) -> ("error out"=w523:errorcluster, "Instrument out"=w525:refnum<class "Inst.TSL210.lvclass">)  [unwired: 6 in]
            n182 = Bundle By Name(cluster=w527, "Instrument"=w525) -> (w528:T8)
            n183 = call <vilib>:"Add State(s) to Queue__jki_lib_state_machine.vi"("State(s) in Front (\"\")"="" ("State(s) in Front (\"\")"), "State(s) in (\"\")"=w532) -> ("States Out"=w531:string)  [unwired: 13 in]
          }
          frame "Action: Laser Toggle" {
            # "Send a message (command, data, etc) to the Instrument:process.vi"
            n184 = Unbundle By Name(w539) -> ("Instrument"=w538:refnum<class "Inst.TSL210.lvclass">)
            n185 = call <userlib>:"Instrument.MessageToProcess.vi"("error in (no error)"=w536, "Data"="LD", "Command"="Laser Toggle", "Instrument"=w538) -> ("error out"=w535:errorcluster, "Instrument out"=w537:refnum<class "Inst.TSL210.lvclass">)  [unwired: 6 in]
            n186 = Bundle By Name(cluster=w539, "Instrument"=w537) -> (w540:T8)
            n187 = call <vilib>:"Add State(s) to Queue__jki_lib_state_machine.vi"("State(s) in Front (\"\")"="" ("State(s) in Front (\"\")"), "State(s) in (\"\")"=w544) -> ("States Out"=w543:string)  [unwired: 13 in]
          }
          frame "Action: Coherence Toggle" {
            # "Send a message (command, data, etc) to the Instrument:process.vi"
            n188 = Unbundle By Name(w551) -> ("Instrument"=w550:refnum<class "Inst.TSL210.lvclass">)
            n189 = call <userlib>:"Instrument.MessageToProcess.vi"("error in (no error)"=w548, "Data"="COH", "Command"="Coherence Toggle", "Instrument"=w550) -> ("error out"=w547:errorcluster, "Instrument out"=w549:refnum<class "Inst.TSL210.lvclass">)  [unwired: 6 in]
            n190 = Bundle By Name(cluster=w551, "Instrument"=w549) -> (w552:T8)
            n191 = call <vilib>:"Add State(s) to Queue__jki_lib_state_machine.vi"("State(s) in Front (\"\")"="" ("State(s) in Front (\"\")"), "State(s) in (\"\")"=w556) -> ("States Out"=w555:string)  [unwired: 13 in]
          }
          frame "Action: ACC Toggle" {
            # "Send a message (command, data, etc) to the Instrument:process.vi"
            n192 = Unbundle By Name(w563) -> ("Instrument"=w562:refnum<class "Inst.TSL210.lvclass">)
            n193 = call <userlib>:"Instrument.MessageToProcess.vi"("error in (no error)"=w560, "Data"="ACC", "Command"="ACC Toggle", "Instrument"=w562) -> ("error out"=w559:errorcluster, "Instrument out"=w561:refnum<class "Inst.TSL210.lvclass">)  [unwired: 6 in]
            n194 = Bundle By Name(cluster=w563, "Instrument"=w561) -> (w564:T8)
            n195 = call <vilib>:"Add State(s) to Queue__jki_lib_state_machine.vi"("State(s) in Front (\"\")"="" ("State(s) in Front (\"\")"), "State(s) in (\"\")"=w568) -> ("States Out"=w567:string)  [unwired: 13 in]
          }
          frame "Action: Send Message to Child" {
            # "Send a message (command, data, etc) to the Instrument.Child:process.vi"
            n196 = Unbundle By Name(w573) -> ("Instrument"=w572:refnum<class "Inst.TSL210.lvclass">)  [unwired: 1 out]
            n197 = call "Inst.TSL210.MessageToProcess.vi"("error in (no error)"=w570, "Inst.TSL210 in"=w572) -> ("error out"=w569:errorcluster, "Inst.TSL210 out"=w571:refnum<class "Inst.TSL210.lvclass">)  [unwired: 8 in]
            n198 = Bundle By Name(cluster=w573, "Instrument"=w571) -> (w574:T8)
            n199 = call <vilib>:"Add State(s) to Queue__jki_lib_state_machine.vi"("State(s) in Front (\"\")"="" ("State(s) in Front (\"\")"), "State(s) in (\"\")"=w578) -> ("States Out"=w577:string)  [unwired: 13 in]
          }
        }
      }
    }
    frame Error {
    }
  }
  n200 = call-parent "Process.vi"("error in"=w5, "Instrument UI in"=w4) -> ("error out"=w2:errorcluster, "Instrument UI out"=→"Inst UI.TSL210 out":refnum<class "Inst UI.TSL210.lvclass">)  [unwired: 8 in]
  n201 = Merge Errors(w2, w1) -> (→"error out":errorcluster)
